vi "Initialize.vi"(5 "TCP Configuration":T1, 6 "Baud Rate Override":u32, 7 "Serial Port":refnum<visa-resource-name>="N/A", 8 "Error In":errorcluster, 10 "Interface":T2, 11 "IO":T7) -> (0 "Error Out":errorcluster, 2 "Device Name":string, 3 "LINX Resource":T3={"IO"=enum."Remote", "Interface"=enum."Serial", "LINX Device Config"={"Interface"=enum."Serial", "COM Port"="COM13", "TCP Configuration"={"IP Address"="", "Port"=0}, "Device Family"=1, "Device ID"=1, "Device Name"="myRIO-1900", "TCP Ref"=refnum, "Channels"={"DI"=[0, 1, 2, 3, 4, 5, 6, 7, 8, 9, 10, 11, 12, 13, 14, 15, 16, 17, 18, 19, 20, 21, 22, 23, 24, 25, 26, 27, 28, 29, 30, 31, 32, 33, 34, 35, 36, 37, 38, 39, 40, 41, 42, 43, 44, 45, 46], "DO"=[0, 1, 2, 3, 4, 5, 6, 7, 8, 9, 10, 11, 12, 13, 14, 15, 16, 17, 18, 19, 20, 21, 22, 23, 24, 25, 26, 27, 28, 29, 30, 31, 32, 33, 34, 35, 36, 37, 38, 39, 40, 41, 42, 43, 44, 45, 46], "AI"=[0, 1, 2, 3, 4, 5, 6, 7, 8, 9, 10, 11], "AO"=[], "PWM"=[3, 5, 6, 9, 10], "QE"=[], "UART"=[0, 1], "I2C 2"=[0], "SPI"=[0], "CAN"=[], "Servo"=[], "AI Ref (V)"=0.0, "AI Resolution (Bits)"=0, "AO Ref (V)"=0.0, "AO Resolution (Bits)"=0}}})   [LabVIEW 2020, in "LMH-LINX.lvlib"]
doc: "Start a LINX session with programmatically configurable I/O settings. This mode is useful for overrideing the LINX Open VI's default behaviour."
uses:
  LMH-LINX.lvlib
  Private/Type Defs/User Platform.ctl
  Private/Type Defs/LINX Ref.ctl
  Private/Type Defs/Platform.ctl
  Private/Type Defs/Interface.ctl
  Private/Device/Type Defs/LINX Device Config.ctl
  Private/Device/Type Defs/TCP Config.ctl
  Private/Device/Type Defs/Channels.ctl
  Private/Utilties/Generate Error.vi
  Private/Local IO/Utilities/Load Device Info.vi
  Private/Local IO/Utilities/Load Device Channels.vi
  Private/Device/Device.lvlib
  Private/Local IO/Local IO.lvlib
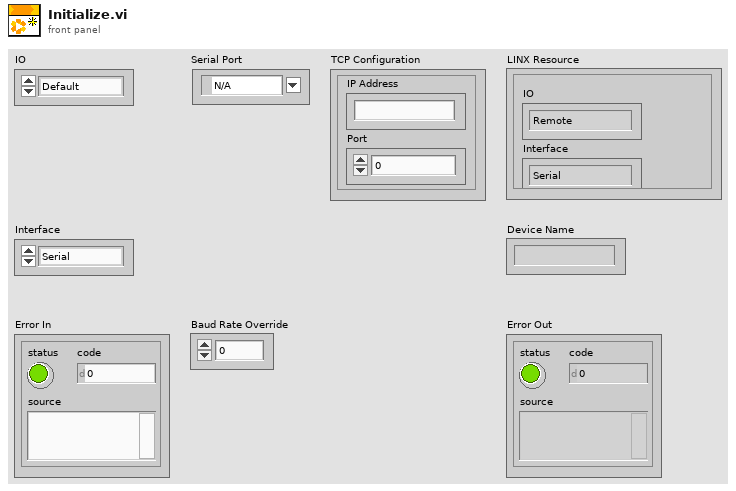
[diagram p1: front panel]
types:
  T1 = typedef "LMH-LINX.lvlib/Device.lvlib/TCP Config.ctl" = cluster{"IP Address":string, "Port":u16}
  T2 = typedef "LMH-LINX.lvlib/Interface.ctl" = enum16{"Serial", "TCP"}
  T3 = typedef "LMH-LINX.lvlib/LINX Ref.ctl" = cluster{"IO":T4, "Interface":T2, "LINX Device Config":T5}
  T4 = typedef "LMH-LINX.lvlib/Platform.ctl" = enum16{"Remote", "Local"}
  T5 = typedef "LMH-LINX.lvlib/Device.lvlib/LINX Device Config.ctl" = cluster{"Interface":T2, "COM Port":refnum<visa-resource-name>, "TCP Configuration":T1, "Device Family":u8, "Device ID":u8, "Device Name":string, "TCP Ref":refnum<k5>, "Channels":T6}
  T6 = typedef "LMH-LINX.lvlib/Channels.ctl" = cluster{"DI":u8[], "DO":u8[], "AI":u8[], "AO":u8[], "PWM":u8[], "QE":u8[], "UART":u8[], "I2C 2":u8[], "SPI":u8[], "CAN":u8[], "Servo":u8[], "AI Ref (V)":dbl, "AI Resolution (Bits)":u8, "AO Ref (V)":dbl, "AO Resolution (Bits)":u8}
  T7 = typedef "LMH-LINX.lvlib/User Platform.ctl" = enum16{"Default", "Remote", "Local"}
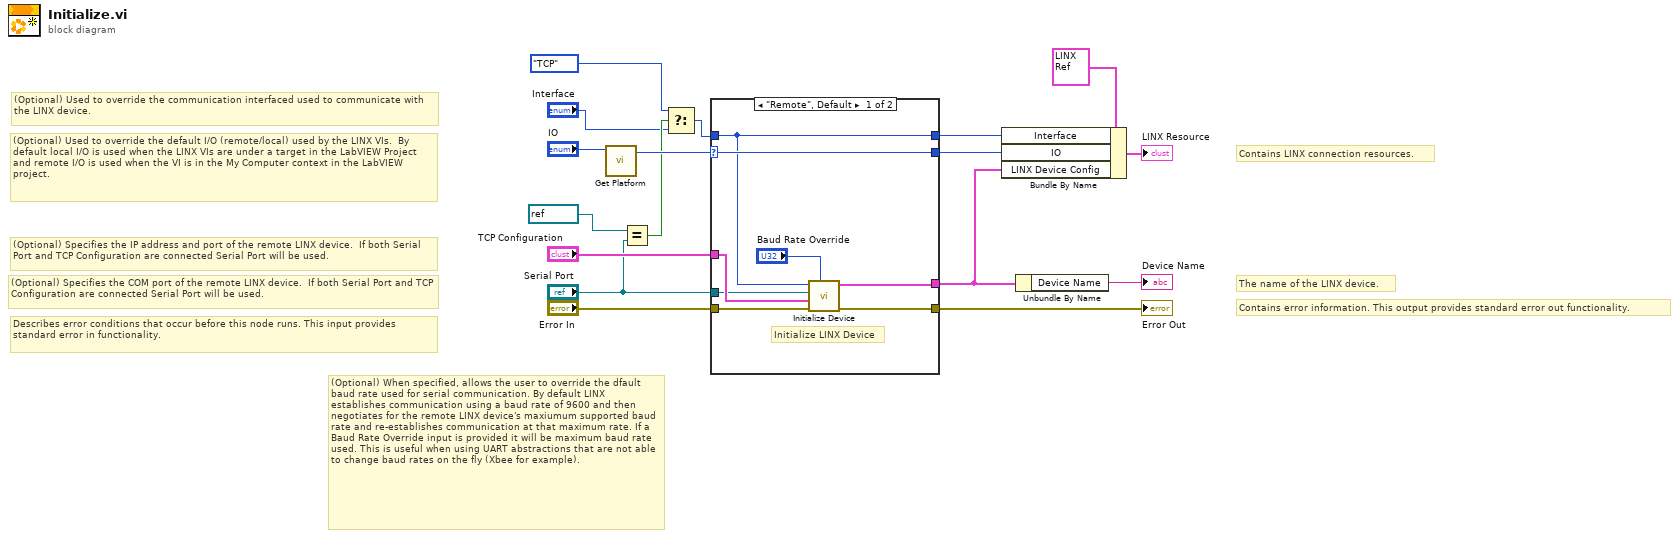
[diagram p0: block diagram]
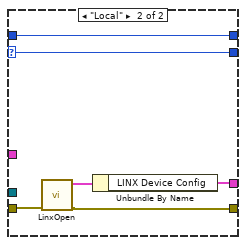
[diagram p2: hidden frame]
diagram:
  # "(Optional) Used to override the default I/O (remote/local) used by the LINX VIs.  By default local I/O is used when the LINX VIs are under a target in the LabVIEW Project and remote I/O is used when the VI is in the My Computer context in the LabVIEW project."
  # "(Optional) Used to override the communication interfaced used to communicate with the LINX device."
  # "(Optional) Specifies the IP address and port of the remote LINX device.  If both Serial Port and TCP Configuration are connected Serial Port will be used."
  # "(Optional) When specified, allows the user to override the dfault baud rate used for serial communication. By default LINX establishes communication using a baud rate of 9600 and then negotiates for the remote LINX device's maxiumum supported baud rate and re-establishes communication at that maximum rate. If a Baud Rate Override input is provided it will be maximum baud rate used. This is useful when using UART abstractions that are not able to change baud rates on the fly (Xbee for example)."
  # "(Optional) Specifies the COM port of the remote LINX device.  If both Serial Port and TCP Configuration are connected Serial Port will be used."
  # "Describes error conditions that occur before this node runs. This input provides standard error in functionality."
  # "Contains LINX connection resources."
  # "The name of the LINX device."
  # "Contains error information. This output provides standard error out functionality."
  n1 = call "Get Platform.vi"("IO"="IO") -> ("IO"=w15:T4)  [unwired: 10 in]
  n2 = Equal?(x=refnum<visa-resource-name> "N/A", y="Serial Port") -> (x = y?=w4:bool)
  n3 = Select(t=Interface."TCP" ("f"), s=w4, f="Interface") -> (s? t:f=w3:T2)
  n4 = case shown="\"Remote\", Default" w15 {
    selector: w15 -> [w25 w31]
    tunnel: [w22 w26] -> w8
    tunnel: [w23 w28] -> w13
    tunnel: "Error In" -> [w24 w29]
    tunnel: [w25 w31] -> w10
    tunnel: "Serial Port" -> [w20 _]
    tunnel: w3 -> [w19 w30]
    tunnel: "TCP Configuration" -> [w21 _]
    tunnel: [w19 w30] -> w9
    frame "Remote", Default {
      # "Initialize LINX Device"
      n5 = call "Initialize Device.vi"("Baud Rate Override"="Baud Rate Override", "Error In"=w24, "TCP Configuration"=w21, "COM Port"=w20, "Interface"=w19) -> ("Error Out"=w23:errorcluster, "LINX Device Config"=w22:T5)  [unwired: 5 in]
    }
    frame "Local" {
      n6 = call "LinxOpen.vi"("Error In"=w29) -> ("Error Out"=w28:errorcluster, "LINX Resource"=w27:T3)  [unwired: 9 in]
      n7 = Unbundle By Name(w27) -> ("LINX Device Config"=w26:T5)
    }
  }
  "Error Out" <- w13
  n8 = Bundle By Name(cluster=T3 {"IO"=enum."Remote", "Interface"=enum."Serial", "LINX Device Config"={"Interface"=enum."Serial", "COM Port"="", "TCP Configuration"={"IP Address"="", "Port"=0}, "Device Family"=0, "Device ID"=0, "Device Name"="", "TCP Ref"=refnum, "Channels"={"DI"=[], "DO"=[], "AI"=[], "AO"=[], "PWM"=[], "QE"=[], "UART"=[], "I2C 2"=[], "SPI"=[], "CAN"=[], "Servo"=[], "AI Ref (V)"=0.0, "AI Resolution (Bits)"=0, "AO Ref (V)"=0.0, "AO Resolution (Bits)"=0}}} ("LINX Resource"), "Interface"=w9, "IO"=w10, "LINX Device Config"=w8) -> (→"LINX Resource":T3)
  n9 = Unbundle By Name(w8) -> ("Device Name"=→"Device Name":string)
